vi "XML Script - GenericSubVI (String).vi"(0 "name":string, 1 "prefix (name)":string, 2 "path":string, 3 "instantiationPath":string, 5 "in":i32=-1, 8 "out":i32=-1) -> (6 "XML Script Command - SubVI":string, 9 "name (wire source)":string)   [LabVIEW 2017]
uses:
  <vilib>/_script/XML Scripting/XML Script Tag.ctl
  <vilib>/_script/XML Scripting/XML Script Attribute.ctl
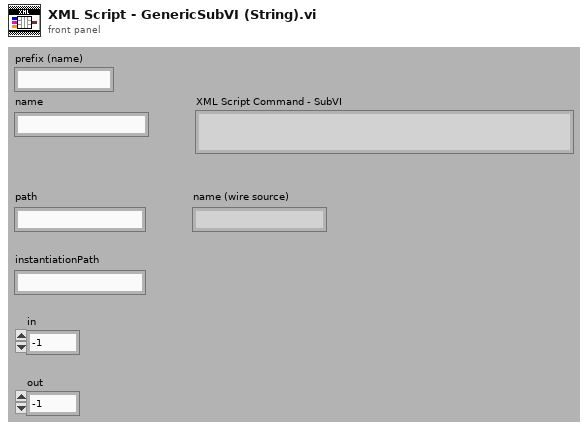
[diagram p1: front panel]
types:
  T1 = typedef "XML Script Attribute.ctl" = enum16{"name", "style", "path", "position", "in", "out", "width", "height", "index", "value", "default", "location", "offset", "typeindex", "size", "source", "destination", "indicator", "type", "controlname", "label", "conpaneidx", "mode", "description", "hasCondTerm", "linkIdentity", "caseselectortype", "concatInputs", "inName", "instantiationpath", "loopCondition", "IndexMode", "formulaInputs", "formulaOutputs", "msnFuncName", "msnIsDynamic", "msnIsODEUserFunction", "ignoreSearchDialog"}
  T2 = typedef "XML Script Tag.ctl" = enum16{"Script", "Function", "SubVI", "GrowableFunction", "Structure", "MultiframeStructure", "Frame", "Tunnel", "ShiftRegister", "Constant", "Control", "Terminal", "Wire", "StaticVIReference", "ControlTerminal", "CompoundArithmetic", "FlatSequence", "FlatSequenceFrame", "MathScriptCallByRef", "BuildArray", "GenericSubVI", "MathScriptNode"}
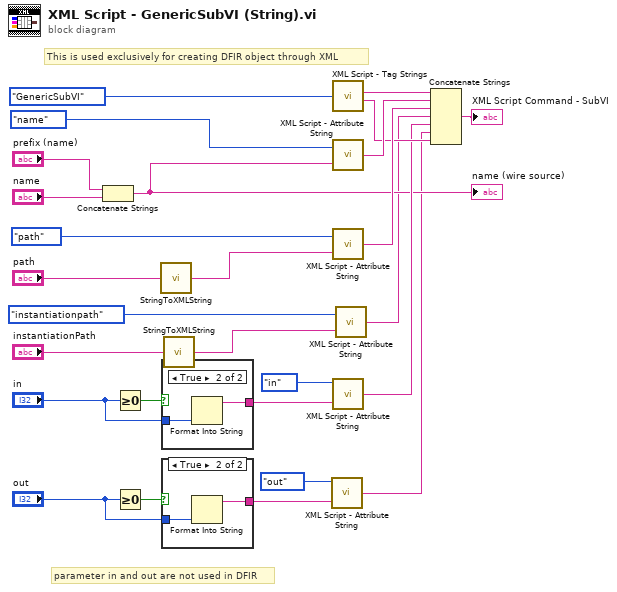
[diagram p0: block diagram]
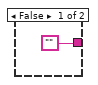
[diagram p2: hidden frame]
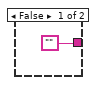
[diagram p3: hidden frame]
diagram:
  # "parameter in and out are not used in DFIR"
  # "This is used exclusively for creating DFIR object through XML"
  n1 = Concatenate Strings("prefix (name)", "name") -> (w12:string)
  "name (wire source)" <- w12
  n2 = Greater Or Equal To 0?(x="in") -> (x >= 0?=w17:bool)
  n3 = Greater Or Equal To 0?(x="out") -> (x >= 0?=w4:bool)
  n4 = call <vilib>:"StringToXMLString.vi"("String"="path") -> ("Valid XML String (out)"=w10:string)
  n5 = case shown="True" w17 {
    tunnel: "in" -> [_ w30]
    tunnel: ["" w29] -> w19
    frame False {
    }
    frame True {
      n6 = Format Into String(w30) -> (resulting string=w29:string)  [unwired: 3 in, 1 out]
    }
  }
  n7 = case shown="True" w4 {
    tunnel: "out" -> [_ w33]
    tunnel: ["" w32] -> w2
    frame False {
    }
    frame True {
      n8 = Format Into String(w33) -> (resulting string=w32:string)  [unwired: 3 in, 1 out]
    }
  }
  n9 = call <vilib>:"StringToXMLString.vi"("String"="instantiationPath") -> ("Valid XML String (out)"=w9:string)
  n10 = call <vilib>:"XML Script - Attribute String.vi"("Attribute String"=w2, "XML Script Attribute"=XML_Script_Attribute."out") -> ("XML Script - Attribute String"=w1:string)
  n11 = call <vilib>:"XML Script - Tag Strings.vi"("XML Script Tag"=XML_Script_Tag."GenericSubVI") -> ("XML String - Begin Tag"=w25:string, "XML String - End Tag"=w20:string)  [unwired: 2 out]
  n12 = call <vilib>:"XML Script - Attribute String.vi"("Attribute String"=w12, "XML Script Attribute"=XML_Script_Attribute."name") -> ("XML Script - Attribute String"=w23:string)
  n13 = call <vilib>:"XML Script - Attribute String.vi"("Attribute String"=w10, "XML Script Attribute"=XML_Script_Attribute."path") -> ("XML Script - Attribute String"=w21:string)
  n14 = call <vilib>:"XML Script - Attribute String.vi"("Attribute String"=w19, "XML Script Attribute"=XML_Script_Attribute."in") -> ("XML Script - Attribute String"=w15:string)
  n15 = call <vilib>:"XML Script - Attribute String.vi"("Attribute String"=w9, "XML Script Attribute"=XML_Script_Attribute."instantiationpath") -> ("XML Script - Attribute String"=w6:string)
  n16 = Concatenate Strings(w25, w23, w21, w6, w15, w1, w20) -> (→"XML Script Command - SubVI":string)
